vi "PH_BackreflectionMeas.Set Default.vi"(0 "i ref in":refnum<vi>, 5 "error in":errorcluster) -> (14 "i ref out":refnum<vi>, 19 "error out":errorcluster)   [LabVIEW 2014, in "PH_BackreflectionMeas.lvlib"]
doc: "This VI reads the default configuration from the data base and sets the hardware."
uses:
  PH_BackreflectionMeas.lvlib
  PH_Devices/PH_TKTDS-30xx/PH_TKTDS-30xx.lvlib
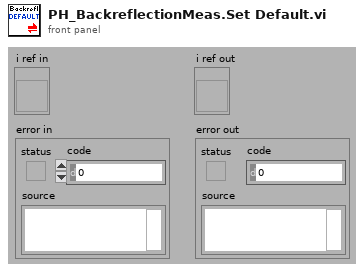
[diagram p1: front panel]
types:
  T1 = typedef "PH_TKTDS-30xx.lvlib/PH_TKTDS-30xx.i attribute.ctl" = cluster{"Default VISA Resource":string, "VISA Resource Name":refnum<visa-resource-name>, "Revision":cluster{"Instrument Driver":string, "Instrument Firmware":string}, "Selftest":cluster{"Result":u32, "Message":string}, "Channels":T2[], "Trigger Configuration":T3, "Acquisition Configuration":T4, "Fetched Waveforms":T5[], "GUI Refs":T6, "GUI Refs Channels":refnum<vi>[], "State":T7, "Error Message":string, "Allow Prdc Loop?":bool}
  T2 = typedef "PH_TKTDS-30xx.lvlib/PH_TKTDS-30xx.Channel Config.ctl" = cluster{"Channel Name":string, "Input Impedance":string, "Max Input Frequency":string, "Vertical Coupling":i32, "Channel Enabled":bool, "Probe Attenuation":dbl, "Vertical Range":dbl, "Vertical Offset":dbl}
  T3 = typedef "PH_TKTDS-30xx.lvlib/PH_TKTDS-30xx.Trigger Config.ctl" = cluster{"Source":string, "Slope":i32, "Level [V]":dbl}
  T4 = typedef "PH_TKTDS-30xx.lvlib/PH_TKTDS-30xx.Acquisition Config.ctl" = cluster{"Time base":dbl, "Record Length":u16, "Start Time":dbl, "Type":i32, "Continuous":bool}
  T5 = typedef "PH_TKTDS-30xx.lvlib/PH_TKTDS-30xx.fetched Waveform.ctl" = cluster{"Source":string, "Actual Points":u32, "Initial X":dbl, "X Increment":dbl, "Waveform Array":dbl[]}
  T6 = typedef "PH_TKTDS-30xx.lvlib/PH_TKTDS-30xx.GUI Refs.ctl" = cluster{"Trigger":refnum<vi>, "Acquisition":refnum<vi>, "Graph":refnum<vi>, "State":refnum<vi>, "Delete":refnum<vi>, "Channel to be positioned":refnum<vi>, "Postion":refnum<vi>, "Display Intensity":refnum<vi>, "VISA Resource":refnum<vi>}
  T7 = typedef "PH_StatusHandler.lvlib/PH_StatusHandler.Status.ctl" = i16
  T8 = typedef "PH_BackreflectionMeas.lvlib/PH_BackreflectionMeas.i attribute.ctl" = cluster{"GUI Refs":cluster{"Get Data":refnum<vi>, "BR State":refnum<vi>, "Reset warning":refnum<vi>, "Low Energy Graph":refnum<vi>}, "Status":cluster{"Reset Warning":bool}, "Default Low Energy Chan Settings":T2, "Default High Energy Chan Settings":T2, "Default Trigger Settings":T3, "Default Acqu Settings":T4, "Limit [V]":dbl}
  T9 = cluster{"Label.Text":string, "Default High Energy Chan Settings":T2}
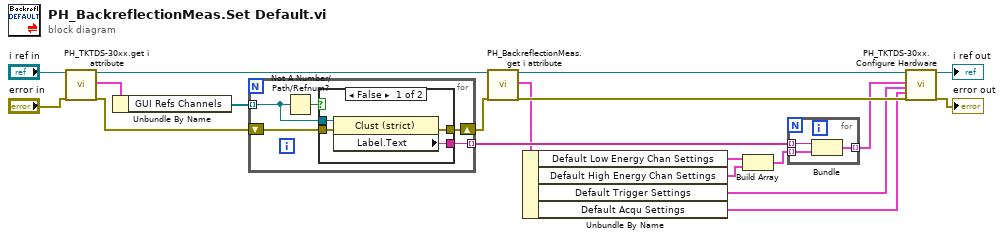
[diagram p0: block diagram]
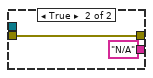
[diagram p2: hidden frame]
diagram:
  n1 = call "PH_TKTDS-30xx.get i attribute.vi"("i ref in"="i ref in", "error in (no error)"="error in") -> ("i ref out"=w15:refnum<vi>, "i attribute"=w14:T1, "error out"=w9:errorcluster)  [unwired: 15 in]
  n2 = Unbundle By Name(w14) -> ("GUI Refs Channels"=w13:refnum<vi>[])
  n3 = for {
    shift-right: [w23] -> w8
    shift-left: w9 -> [w24]
    tunnel: [w22] -> w12 mode=indexing
    tunnel: w13 -> [w20] mode=indexing
    n4 = Not A Number/Path/Refnum?(number/path/refnum=w20) -> (NaN/Path/Refnum?=w21:bool)
    n5 = case shown="False" w21 {
      tunnel: w24 -> [w28 w30]
      tunnel: [w27 w30] -> w23
      tunnel: [w26 "N/A" ("Label.Text")] -> w22
      tunnel: w20 -> [w25 _]
      frame False {
        n6 = property class="Clust (strict)"(reference=w25, error in=w28) -> (error out=w27:errorcluster, "Label.Text"=w26:string)  [unwired: 1 out]
      }
      frame True {
      }
    }
  }
  n7 = call "PH_BackreflectionMeas.get i attribute.vi"("i ref in"=w15, "error in (no error)"=w8) -> ("i ref out"=w19:refnum<vi>, "i attribute"=w5:T8, "error out"=w18:errorcluster)  [unwired: 15 in]
  n8 = Unbundle By Name(w5) -> ("Default Low Energy Chan Settings"=w1:T2, "Default High Energy Chan Settings"=w2:T2, "Default Trigger Settings"=w3:T3, "Default Acqu Settings"=w4:T4)
  n9 = Build Array(w1, w2) -> (w17:T2[])
  n10 = for {
    tunnel: w17 -> [w33] mode=indexing
    tunnel: w12 -> [w32] mode=indexing
    tunnel: [w31] -> w16 mode=indexing
    n11 = Bundle("Label.Text"=w32, "Default High Energy Chan Settings"=w33) -> (w31:T9)  [unwired: 1 in]
  }
  n12 = call "PH_TKTDS-30xx.Configure Hardware.vi"("i ref in"=w19, "Channels Sets"=w16, "Trigger Settings"=w3, "Acqu Settings"=w4, "error in"=w18) -> ("i ref out"=→"i ref out":refnum<vi>, "error out"=→"error out":errorcluster)  [unwired: 13 in]
